vi "calculate_coolprop.vi"(4 "InputCode":T2(ring), 5 "error in":errorcluster, 6 "Input_2":dbl=-1111111111.0 format="%#.6f", 7 "Input_1":dbl=-1111111111.0 format="%#.6f", 8 "Common In":T1={"units"=enum."SI", "Coolprop Directory"=path "C:/Labview/Libfolder/CoolProp.dll", "FluidName"="Water", "Molecular mass [kg/kmol]"=0.0, "Quality [-]"=0.0, "Temperature [°C]"=0.0, "Pressure [bar]"=0.0, "Density [kg/m3]"=0.0, "Spec. heat - ideal gas @ cst. pressure [kJ/kg]"=0.0, "Spec. heat @ cst. pressure [kJ/kg]"=0.0, "Spec. heat @ cst. volume [kJ/kg]"=0.0, "Internal energy [ kJ/kg]"=0.0, "Enthalpy [kJ/kg]"=0.0, "Entropy [kJ/kg-K]"=0.0, "Speed of sound [m/s]"=0.0, "Gibbs function [kJ/kg]"=0.0, "Dynamic viscosity [Pa-s]"=0.0, "Thermal conductivity [kW/m-K]"=0.0, "Surface Tension [N/m]"=0.0, "Accentric factor [-]"=0.0}) -> (0 "error out":errorcluster, 3 "Common Out":T1)   [LabVIEW 2017]
doc: "Calculates thermodynamic values of a certain point for the given fluid, gathered in \"Common Out\".\nCommon connection and InputCode are required.\nIf an input value remains unconnected, the corresponding value in the common will be used.\n\nInput_1 corresponds with the first parameter chosen with the input code.\nInput_2 corresponds with the second parameter chosen with the input code.\ne.g.: if input code is \"TP\", Input_1 requires a temperature (°C) and Input_2 required a pressure (bar)\n\n---\nDesigned by Department of Industrial System and Product Design, Ghent University.\nContact: sergei.gusev@ugent.be; jan.nolens@ugent.be\n\nBased on a Labview-Refprop Wrapper downloaded from Nist.org\nMore info: ken_pop@tom.com yan.ding@jci.com"
uses:
  FluidCommon.ctl
panel:
  out "Array":dbl[](array[numeric])
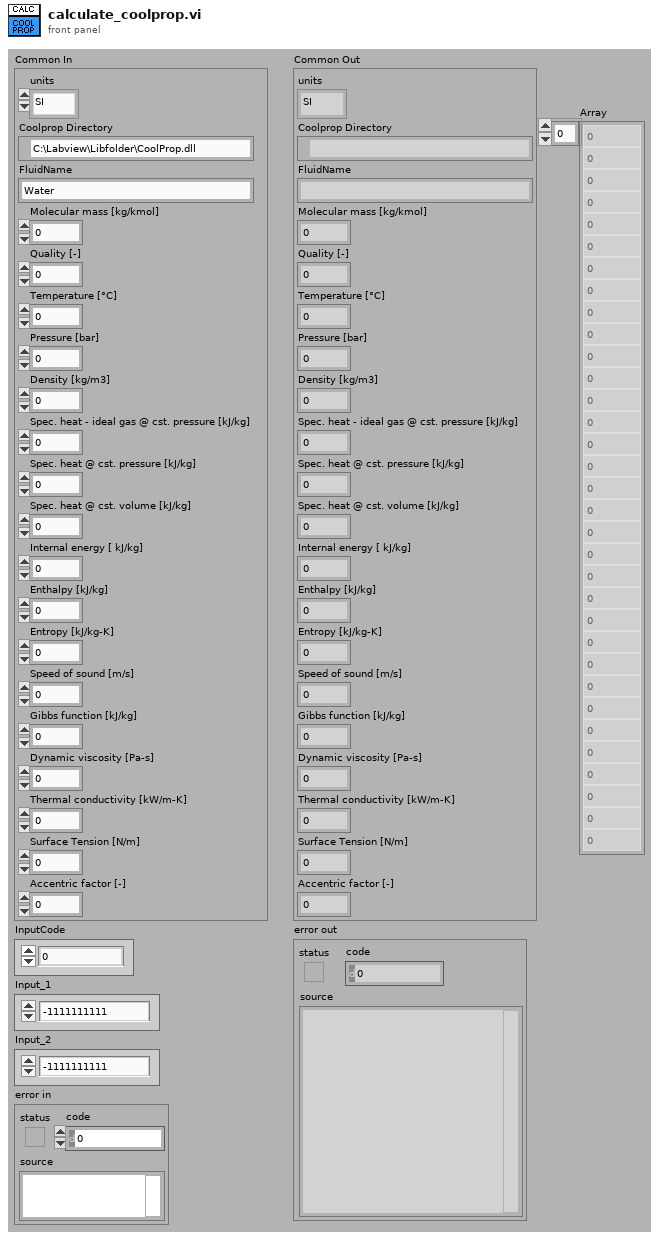
[diagram p1: front panel]
types:
  T1 = typedef "FluidCommon.ctl" = cluster{"units":enum16{"SI", "IP"}, "Coolprop Directory":path, "FluidName":string, "Molecular mass [kg/kmol]":dbl, "Quality [-]":dbl, "Temperature [°C]":dbl, "Pressure [bar]":dbl, "Density [kg/m3]":dbl, "Spec. heat - ideal gas @ cst. pressure [kJ/kg]":dbl, "Spec. heat @ cst. pressure [kJ/kg]":dbl, "Spec. heat @ cst. volume [kJ/kg]":dbl, "Internal energy [ kJ/kg]":dbl, "Enthalpy [kJ/kg]":dbl, "Entropy [kJ/kg-K]":dbl, "Speed of sound [m/s]":dbl, "Gibbs function [kJ/kg]":dbl, "Dynamic viscosity [Pa-s]":dbl, "Thermal conductivity [kW/m-K]":dbl, "Surface Tension [N/m]":dbl, "Accentric factor [-]":dbl}
  T2 = enum16{"0", "TP", "TD", "PD", "TQ", "PQ", "HP", "SP", "SH"}
  T3 = enum16{"P [kPa]", "T [K]", "S [kJ/kg/K]", "H [kJ/kg]"}
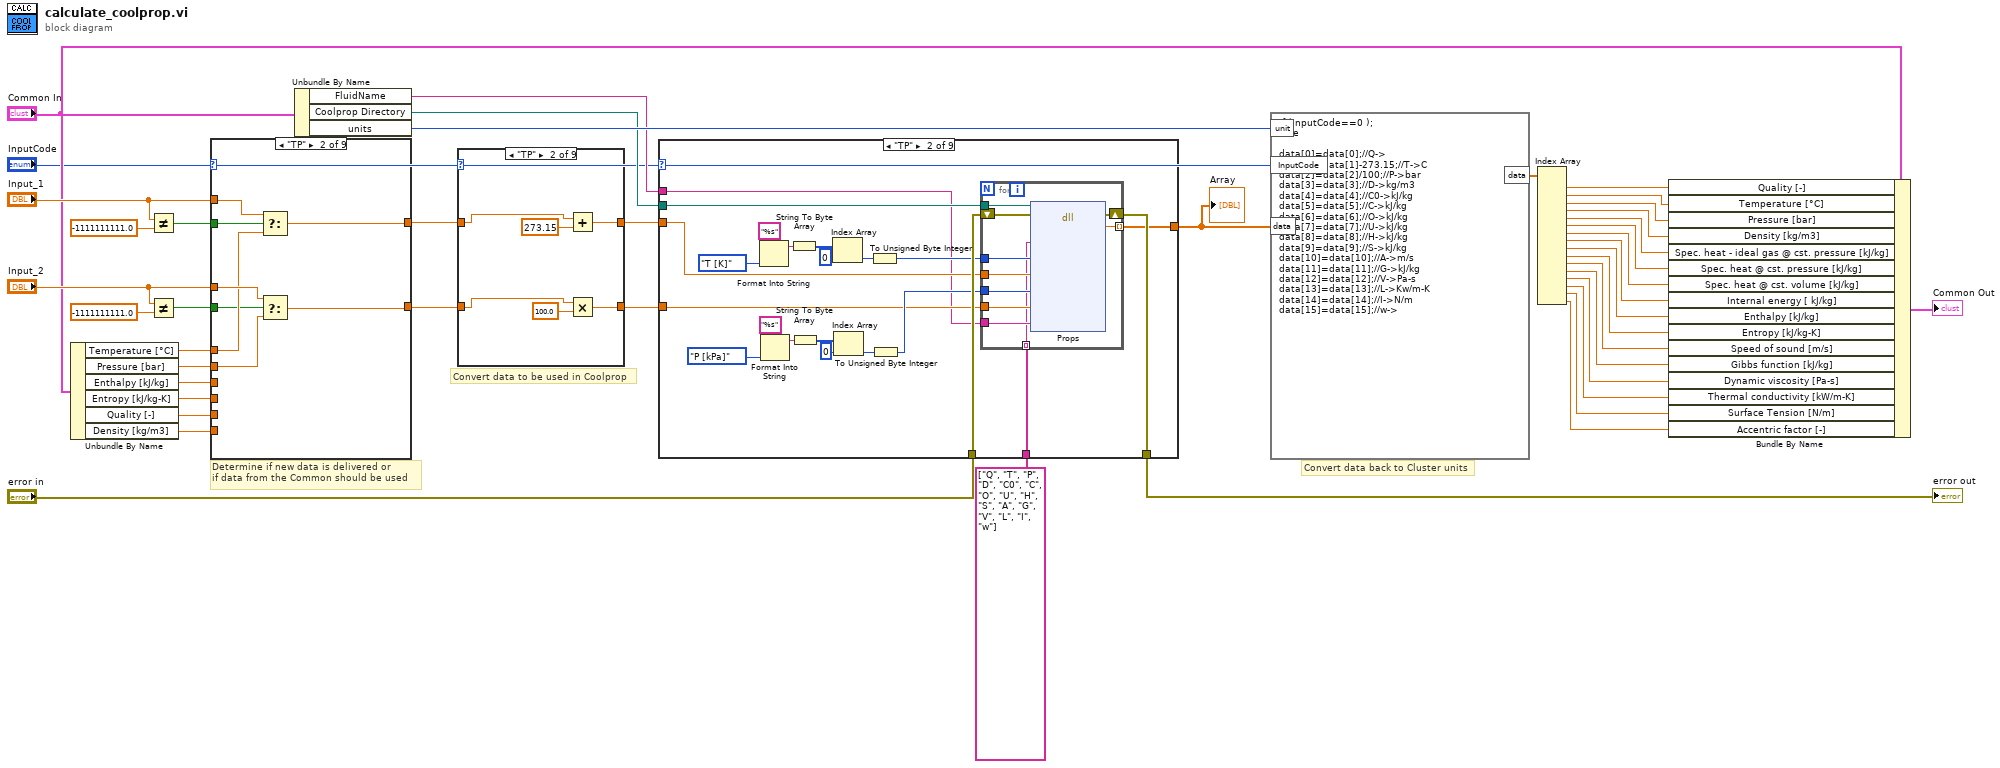
[diagram p0: block diagram]
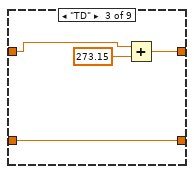
[diagram p3: hidden frame]
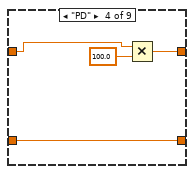
[diagram p4: hidden frame]
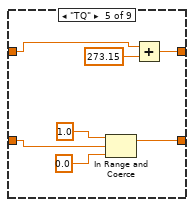
[diagram p5: hidden frame]
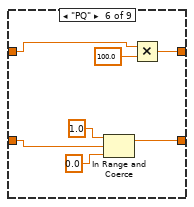
[diagram p6: hidden frame]
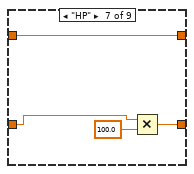
[diagram p7: hidden frame]
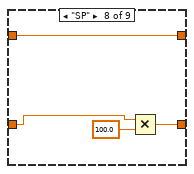
[diagram p8: hidden frame]
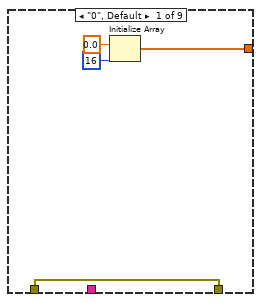
[diagram p10: hidden frame]
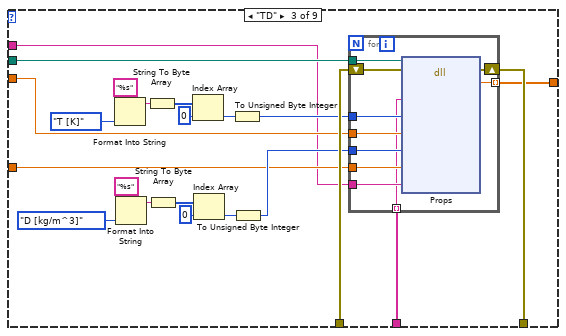
[diagram p11: hidden frame]
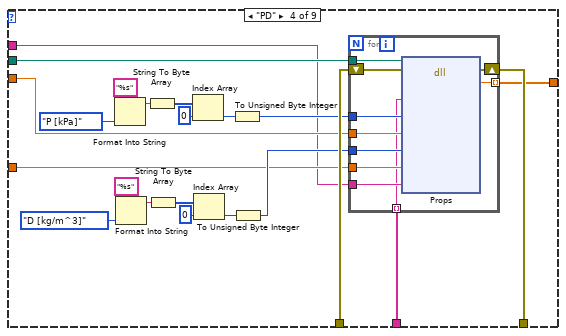
[diagram p12: hidden frame]
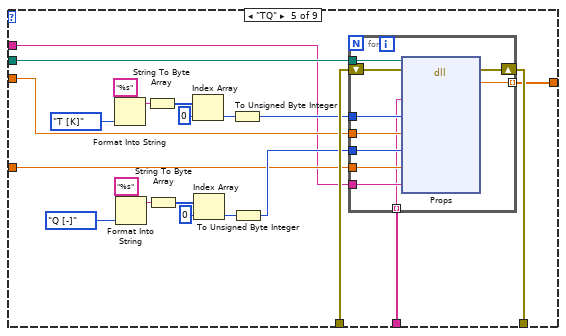
[diagram p13: hidden frame]
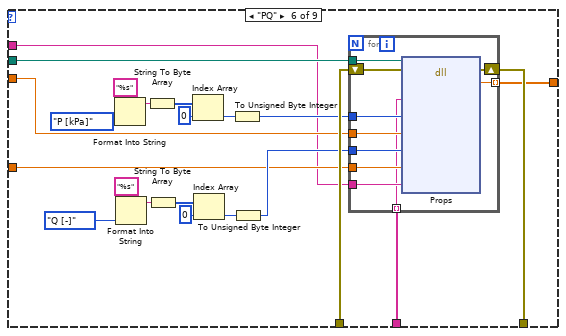
[diagram p14: hidden frame]
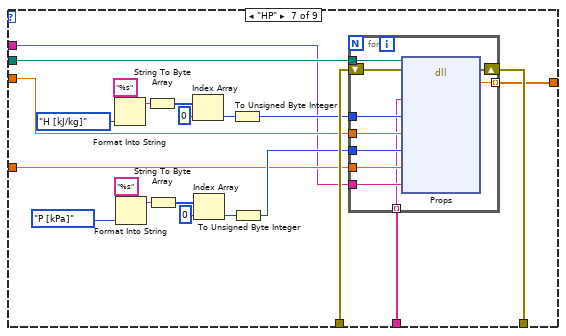
[diagram p15: hidden frame]
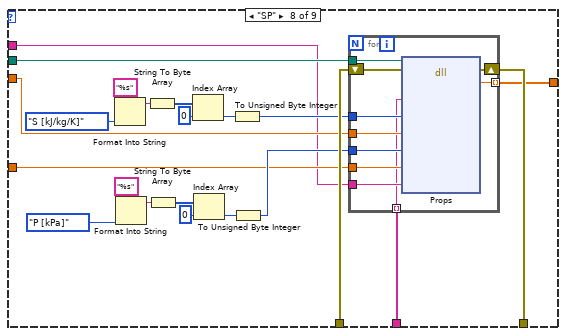
[diagram p16: hidden frame]
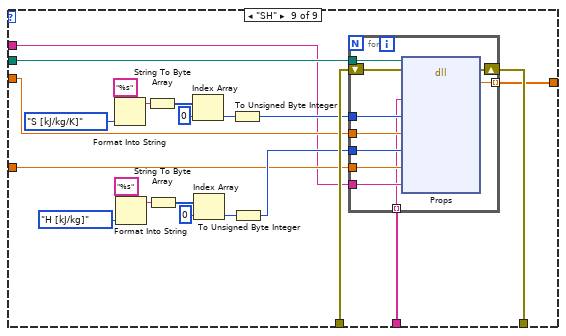
[diagram p17: hidden frame]
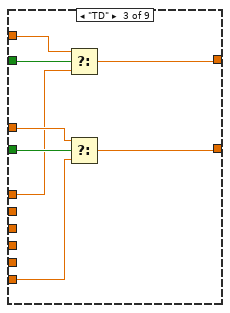
[diagram p19: hidden frame]
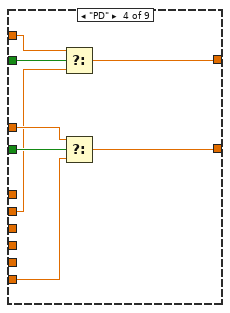
[diagram p20: hidden frame]
diagram:
  # "Convert data back to Cluster units"
  # "Convert data to be used in Coolprop"
  # "Determine if new data is delivered or \nif data from the Common should be used"
  n1 = Unbundle By Name("Common In") -> ("Temperature [°C]"=w35:dbl, "Pressure [bar]"=w34:dbl, "Enthalpy [kJ/kg]"=w33:dbl, "Entropy [kJ/kg-K]"=w32:dbl, "Quality [-]"=w31:dbl, "Density [kg/m3]"=w30:dbl)
  n2 = Not Equal?(x="Input_1", y=-1111111111.0) -> (x != y?=w39:bool)
  n3 = Not Equal?(x="Input_2", y=-1111111111.0) -> (x != y?=w38:bool)
  n4 = case shown="\"TP\"" "InputCode" {
    tunnel: "Input_1" -> [w45 w51 w59 w69 w77 w85 w90 w101 w109]
    tunnel: "Input_2" -> [w44 w53 w57 w67 w75 w83 w92 w99 w107]
    tunnel: w39 -> [_ w49 w58 w68 w76 w84 w91 w100 w108]
    tunnel: w38 -> [_ w48 w56 w66 w74 w82 w93 w98 w106]
    tunnel: w35 -> [_ w50 w55 _ w73 _ _ _ _]
    tunnel: w34 -> [_ w52 _ w65 _ w81 w88 w96 _]
    tunnel: w33 -> [_ _ _ _ _ _ w89 _ w104]
    tunnel: w32 -> [_ _ _ _ _ _ _ w97 w105]
    tunnel: w31 -> [_ _ _ _ w72 w80 _ _ _]
    tunnel: w30 -> [_ _ w54 w64 _ _ _ _ _]
    tunnel: [w45 w47 w60 w62 w70 w78 w86 w94 w102] -> w37
    tunnel: [w44 w46 w61 w63 w71 w79 w87 w95 w103] -> w36
    frame "0", Default {
    }
    frame "TP" {
      n5 = Select(t=w51, s=w49, f=w50) -> (s? t:f=w47:dbl)
      n6 = Select(t=w53, s=w48, f=w52) -> (s? t:f=w46:dbl)
    }
    frame "TD" {
      n7 = Select(t=w59, s=w58, f=w55) -> (s? t:f=w60:dbl)
      n8 = Select(t=w57, s=w56, f=w54) -> (s? t:f=w61:dbl)
    }
    frame "PD" {
      n9 = Select(t=w69, s=w68, f=w65) -> (s? t:f=w62:dbl)
      n10 = Select(t=w67, s=w66, f=w64) -> (s? t:f=w63:dbl)
    }
    frame "TQ" {
      n11 = Select(t=w77, s=w76, f=w73) -> (s? t:f=w70:dbl)
      n12 = Select(t=w75, s=w74, f=w72) -> (s? t:f=w71:dbl)
    }
    frame "PQ" {
      n13 = Select(t=w85, s=w84, f=w81) -> (s? t:f=w78:dbl)
      n14 = Select(t=w83, s=w82, f=w80) -> (s? t:f=w79:dbl)
    }
    frame "HP" {
      n15 = Select(t=w90, s=w91, f=w89) -> (s? t:f=w86:dbl)
      n16 = Select(t=w92, s=w93, f=w88) -> (s? t:f=w87:dbl)
    }
    frame "SP" {
      n17 = Select(t=w101, s=w100, f=w97) -> (s? t:f=w94:dbl)
      n18 = Select(t=w99, s=w98, f=w96) -> (s? t:f=w95:dbl)
    }
    frame "SH" {
      n19 = Select(t=w109, s=w108, f=w105) -> (s? t:f=w102:dbl)
      n20 = Select(t=w107, s=w106, f=w104) -> (s? t:f=w103:dbl)
    }
  }
  n21 = Unbundle By Name("Common In") -> ("FluidName"=w20:string, "Coolprop Directory"=w22:path, "units"=w29:enum16{"SI", "IP"})
  n22 = case shown="\"TP\"" "InputCode" {
    tunnel: [w111 w113 w119 w123 w131 w134 w140 w147 w149] -> w26
    tunnel: w37 -> [w111 w116 w120 w122 w130 w135 w140 w147 w149]
    tunnel: w36 -> [w110 w114 w118 w125 w127 w136 w141 w145 w148]
    tunnel: [w110 w112 w118 w125 w126 w133 w142 w144 w148] -> w25
    frame "0", Default {
    }
    frame "TP" {
      n23 = Add(x=w116, y=273.15) -> (x+y=w113:dbl)
      n24 = Multiply(x=w114, y=100.0 ("x")) -> (x*y=w112:dbl)
    }
    frame "TD" {
      n25 = Add(x=w120, y=273.15) -> (x+y=w119:dbl)
    }
    frame "PD" {
      n26 = Multiply(x=w122, y=100.0 ("x")) -> (x*y=w123:dbl)
    }
    frame "TQ" {
      n27 = In Range and Coerce(upper limit=1.0 ("上限"), x=w127, lower limit=0.0 ("下限")) -> (coerced(x)=w126:dbl)  [unwired: 1 out]
      n28 = Add(x=w130, y=273.15 ("x")) -> (x+y=w131:dbl)
    }
    frame "PQ" {
      n29 = In Range and Coerce(upper limit=1.0 ("上限"), x=w136, lower limit=0.0 ("下限")) -> (coerced(x)=w133:dbl)  [unwired: 1 out]
      n30 = Multiply(x=w135, y=100.0 ("x")) -> (x*y=w134:dbl)
    }
    frame "HP" {
      n31 = Multiply(x=w141, y=100.0 ("x")) -> (x*y=w142:dbl)
    }
    frame "SP" {
      n32 = Multiply(x=w145, y=100.0 ("x")) -> (x*y=w144:dbl)
    }
    frame "SH" {
    }
  }
  n33 = case shown="\"TP\"" "InputCode" {
    tunnel: w26 -> [_ w156 w189 w221 w253 w285 w317 w349 w380]
    tunnel: w25 -> [_ w157 w190 w222 w254 w286 w318 w350 w381]
    tunnel: "error in" -> [w153 w174 w206 w238 w270 w302 w334 w366 w398]
    tunnel: [w153 w173 w205 w237 w269 w301 w333 w365 w397] -> w23
    tunnel: w22 -> [_ w175 w207 w239 w271 w303 w335 w367 w399]
    tunnel: [w150 w172 w204 w236 w268 w300 w332 w364 w396] -> w21
    tunnel: w20 -> [_ w155 w188 w220 w252 w284 w316 w348 w379]
    tunnel: string[] ["Q", "T", "P", "D", "C0", "C", "O", "U", "H", "S", "A", "G", "V", "L", "I", "w"] -> [_ w154 w187 w219 w251 w283 w315 w347 w378]
    frame "0", Default {
      n34 = Initialize Array(0.0 ("元素"), 16 ("维数大小")) -> (w150:dbl[])
    }
    frame "TP" {
      n35 = Format Into String "Format Into String"(format string="%s", T3."T [K]" ("Input Variable #1")) -> (resulting string=w167:string)  [unwired: 2 in, 1 out]
      n36 = Format Into String(format string="%s", T3."P [kPa]" ("Input Variable #1")) -> (resulting string=w161:string)  [unwired: 2 in, 1 out]
      n37 = String To Byte Array(string=w167) -> (unsigned byte array=w169:u8[])
      n38 = String To Byte Array(string=w161) -> (unsigned byte array=w163:u8[])
      n39 = Index Array(array=w169, index=0) -> (element=w171:u8)
      n40 = Index Array(array=w163, index=0) -> (element=w165:u8)
      n41 = To Unsigned Byte Integer(number=w171) -> (unsigned 8bit integer=w159:u8)
      n42 = To Unsigned Byte Integer(number=w165) -> (unsigned 8bit integer=w158:u8)
      n43 = for {
        tunnel: w175 -> [w185]
        shift-right: [w183] -> w173
        shift-left: w174 -> [w184]
        tunnel: [w182] -> w172 mode=indexing
        tunnel: w155 -> [w181]
        tunnel: w157 -> [w180]
        tunnel: w158 -> [w179]
        tunnel: w156 -> [w178]
        tunnel: w159 -> [w177]
        tunnel: w154 -> [w176] mode=indexing
        n44 = dll-call lib="C:/LABVIEW/LibFolder/CoolProp.dll" fn="Props"(path in=w185, error in=w184, "Output"=w176, "Input1"=w177, "Value1"=w178, "Input2"=w179, "Value2"=w180, "Fluid"=w181) -> (error out=w183:errorcluster, "OutputValue"=w182:dbl)  [unwired: 7 in, 1 out]
      }
    }
    frame "TD" {
      n45 = Format Into String "Format Into String"(format string="%s", T3."T [K]" ("Input Variable #1")) -> (resulting string=w199:string)  [unwired: 2 in, 1 out]
      n46 = Format Into String(format string="%s", enum16{"P [kPa]", "Q [-]", "D [kg/m^3]"}."D [kg/m^3]" ("Input Variable #2")) -> (resulting string=w193:string)  [unwired: 2 in, 1 out]
      n47 = String To Byte Array(string=w199) -> (unsigned byte array=w201:u8[])
      n48 = String To Byte Array(string=w193) -> (unsigned byte array=w195:u8[])
      n49 = Index Array(array=w201, index=0) -> (element=w203:u8)
      n50 = Index Array(array=w195, index=0) -> (element=w197:u8)
      n51 = To Unsigned Byte Integer(number=w203) -> (unsigned 8bit integer=w192:u8)
      n52 = To Unsigned Byte Integer(number=w197) -> (unsigned 8bit integer=w191:u8)
      n53 = for {
        tunnel: w207 -> [w217]
        shift-right: [w215] -> w205
        shift-left: w206 -> [w216]
        tunnel: [w214] -> w204 mode=indexing
        tunnel: w188 -> [w213]
        tunnel: w190 -> [w212]
        tunnel: w191 -> [w211]
        tunnel: w189 -> [w210]
        tunnel: w192 -> [w209]
        tunnel: w187 -> [w208] mode=indexing
        n54 = dll-call lib="C:/Coolprop/CoolProp.dll" fn="Props"(path in=w217, error in=w216, "Output"=w208, "Input1"=w209, "Value1"=w210, "Input2"=w211, "Value2"=w212, "Fluid"=w213) -> (error out=w215:errorcluster, "OutputValue"=w214:dbl)  [unwired: 7 in, 1 out]
      }
    }
    frame "PD" {
      n55 = Format Into String "Format Into String"(format string="%s", T3."P [kPa]" ("Input Variable #1")) -> (resulting string=w231:string)  [unwired: 2 in, 1 out]
      n56 = Format Into String(format string="%s", enum16{"P [kPa]", "Q [-]", "D [kg/m^3]"}."D [kg/m^3]" ("Input Variable #2")) -> (resulting string=w225:string)  [unwired: 2 in, 1 out]
      n57 = String To Byte Array(string=w231) -> (unsigned byte array=w233:u8[])
      n58 = String To Byte Array(string=w225) -> (unsigned byte array=w227:u8[])
      n59 = Index Array(array=w233, index=0) -> (element=w235:u8)
      n60 = Index Array(array=w227, index=0) -> (element=w229:u8)
      n61 = To Unsigned Byte Integer(number=w235) -> (unsigned 8bit integer=w224:u8)
      n62 = To Unsigned Byte Integer(number=w229) -> (unsigned 8bit integer=w223:u8)
      n63 = for {
        tunnel: w239 -> [w249]
        shift-right: [w247] -> w237
        shift-left: w238 -> [w248]
        tunnel: [w246] -> w236 mode=indexing
        tunnel: w220 -> [w245]
        tunnel: w222 -> [w244]
        tunnel: w223 -> [w243]
        tunnel: w221 -> [w242]
        tunnel: w224 -> [w241]
        tunnel: w219 -> [w240] mode=indexing
        n64 = dll-call lib="C:/Coolprop/CoolProp.dll" fn="Props"(path in=w249, error in=w248, "Output"=w240, "Input1"=w241, "Value1"=w242, "Input2"=w243, "Value2"=w244, "Fluid"=w245) -> (error out=w247:errorcluster, "OutputValue"=w246:dbl)  [unwired: 7 in, 1 out]
      }
    }
    frame "TQ" {
      n65 = Format Into String "Format Into String"(format string="%s", T3."T [K]" ("Input Variable #1")) -> (resulting string=w263:string)  [unwired: 2 in, 1 out]
      n66 = Format Into String(format string="%s", enum16{"P [kPa]", "Q [-]", "D [kg/m^3]"}."Q [-]" ("Input Variable #2")) -> (resulting string=w257:string)  [unwired: 2 in, 1 out]
      n67 = String To Byte Array(string=w263) -> (unsigned byte array=w265:u8[])
      n68 = String To Byte Array(string=w257) -> (unsigned byte array=w259:u8[])
      n69 = Index Array(array=w265, index=0) -> (element=w267:u8)
      n70 = Index Array(array=w259, index=0) -> (element=w261:u8)
      n71 = To Unsigned Byte Integer(number=w267) -> (unsigned 8bit integer=w256:u8)
      n72 = To Unsigned Byte Integer(number=w261) -> (unsigned 8bit integer=w255:u8)
      n73 = for {
        tunnel: w271 -> [w272]
        shift-right: [w280] -> w269
        shift-left: w270 -> [w281]
        tunnel: [w279] -> w268 mode=indexing
        tunnel: w252 -> [w278]
        tunnel: w254 -> [w277]
        tunnel: w255 -> [w276]
        tunnel: w253 -> [w275]
        tunnel: w256 -> [w274]
        tunnel: w251 -> [w273] mode=indexing
        n74 = dll-call lib="C:/Users/jan.nolens/Desktop/CoolProp.dll" fn="Props"(path in=w272, error in=w281, "Output"=w273, "Input1"=w274, "Value1"=w275, "Input2"=w276, "Value2"=w277, "Fluid"=w278) -> (error out=w280:errorcluster, "OutputValue"=w279:dbl)  [unwired: 7 in, 1 out]
      }
    }
    frame "PQ" {
      n75 = Format Into String "Format Into String"(format string="%s", T3."P [kPa]" ("Input Variable #1")) -> (resulting string=w295:string)  [unwired: 2 in, 1 out]
      n76 = Format Into String(format string="%s", enum16{"P [kPa]", "Q [-]", "D [kg/m^3]"}."Q [-]" ("Input Variable #2")) -> (resulting string=w289:string)  [unwired: 2 in, 1 out]
      n77 = String To Byte Array(string=w295) -> (unsigned byte array=w297:u8[])
      n78 = String To Byte Array(string=w289) -> (unsigned byte array=w291:u8[])
      n79 = Index Array(array=w297, index=0) -> (element=w299:u8)
      n80 = Index Array(array=w291, index=0) -> (element=w293:u8)
      n81 = To Unsigned Byte Integer(number=w299) -> (unsigned 8bit integer=w288:u8)
      n82 = To Unsigned Byte Integer(number=w293) -> (unsigned 8bit integer=w287:u8)
      n83 = for {
        tunnel: w303 -> [w313]
        shift-right: [w311] -> w301
        shift-left: w302 -> [w312]
        tunnel: [w310] -> w300 mode=indexing
        tunnel: w284 -> [w309]
        tunnel: w286 -> [w308]
        tunnel: w287 -> [w307]
        tunnel: w285 -> [w306]
        tunnel: w288 -> [w305]
        tunnel: w283 -> [w304] mode=indexing
        n84 = dll-call lib="C:/Coolprop/CoolProp.dll" fn="Props"(path in=w313, error in=w312, "Output"=w304, "Input1"=w305, "Value1"=w306, "Input2"=w307, "Value2"=w308, "Fluid"=w309) -> (error out=w311:errorcluster, "OutputValue"=w310:dbl)  [unwired: 7 in, 1 out]
      }
    }
    frame "HP" {
      n85 = Format Into String "Format Into String"(format string="%s", T3."H [kJ/kg]" ("Input Variable #1")) -> (resulting string=w327:string)  [unwired: 2 in, 1 out]
      n86 = Format Into String(format string="%s", enum16{"P [kPa]", "Q [-]", "D [kg/m^3]"}."P [kPa]" ("Input Variable #2")) -> (resulting string=w321:string)  [unwired: 2 in, 1 out]
      n87 = String To Byte Array(string=w327) -> (unsigned byte array=w329:u8[])
      n88 = String To Byte Array(string=w321) -> (unsigned byte array=w323:u8[])
      n89 = Index Array(array=w329, index=0) -> (element=w331:u8)
      n90 = Index Array(array=w323, index=0) -> (element=w325:u8)
      n91 = To Unsigned Byte Integer(number=w331) -> (unsigned 8bit integer=w320:u8)
      n92 = To Unsigned Byte Integer(number=w325) -> (unsigned 8bit integer=w319:u8)
      n93 = for {
        tunnel: w335 -> [w345]
        shift-right: [w343] -> w333
        shift-left: w334 -> [w344]
        tunnel: [w342] -> w332 mode=indexing
        tunnel: w316 -> [w341]
        tunnel: w318 -> [w340]
        tunnel: w319 -> [w339]
        tunnel: w317 -> [w338]
        tunnel: w320 -> [w337]
        tunnel: w315 -> [w336] mode=indexing
        n94 = dll-call lib="C:/Coolprop/CoolProp.dll" fn="Props"(path in=w345, error in=w344, "Output"=w336, "Input1"=w337, "Value1"=w338, "Input2"=w339, "Value2"=w340, "Fluid"=w341) -> (error out=w343:errorcluster, "OutputValue"=w342:dbl)  [unwired: 7 in, 1 out]
      }
    }
    frame "SP" {
      n95 = Format Into String "Format Into String"(format string="%s", T3."S [kJ/kg/K]" ("Input Variable #1")) -> (resulting string=w359:string)  [unwired: 2 in, 1 out]
      n96 = Format Into String(format string="%s", enum16{"P [kPa]", "Q [-]", "D [kg/m^3]"}."P [kPa]" ("Input Variable #2")) -> (resulting string=w353:string)  [unwired: 2 in, 1 out]
      n97 = String To Byte Array(string=w359) -> (unsigned byte array=w361:u8[])
      n98 = String To Byte Array(string=w353) -> (unsigned byte array=w355:u8[])
      n99 = Index Array(array=w361, index=0) -> (element=w363:u8)
      n100 = Index Array(array=w355, index=0) -> (element=w357:u8)
      n101 = To Unsigned Byte Integer(number=w363) -> (unsigned 8bit integer=w352:u8)
      n102 = To Unsigned Byte Integer(number=w357) -> (unsigned 8bit integer=w351:u8)
      n103 = for {
        tunnel: w367 -> [w377]
        shift-right: [w375] -> w365
        shift-left: w366 -> [w376]
        tunnel: [w374] -> w364 mode=indexing
        tunnel: w348 -> [w373]
        tunnel: w350 -> [w372]
        tunnel: w351 -> [w371]
        tunnel: w349 -> [w370]
        tunnel: w352 -> [w369]
        tunnel: w347 -> [w368] mode=indexing
        n104 = dll-call lib="C:/Coolprop/CoolProp.dll" fn="Props"(path in=w377, error in=w376, "Output"=w368, "Input1"=w369, "Value1"=w370, "Input2"=w371, "Value2"=w372, "Fluid"=w373) -> (error out=w375:errorcluster, "OutputValue"=w374:dbl)  [unwired: 7 in, 1 out]
      }
    }
    frame "SH" {
      n105 = Format Into String "Format Into String"(format string="%s", T3."S [kJ/kg/K]" ("Input Variable #1")) -> (resulting string=w391:string)  [unwired: 2 in, 1 out]
      n106 = Format Into String(format string="%s", T3."H [kJ/kg]" ("Input Variable #1")) -> (resulting string=w385:string)  [unwired: 2 in, 1 out]
      n107 = String To Byte Array(string=w391) -> (unsigned byte array=w393:u8[])
      n108 = String To Byte Array(string=w385) -> (unsigned byte array=w387:u8[])
      n109 = Index Array(array=w393, index=0) -> (element=w395:u8)
      n110 = Index Array(array=w387, index=0) -> (element=w389:u8)
      n111 = To Unsigned Byte Integer(number=w395) -> (unsigned 8bit integer=w383:u8)
      n112 = To Unsigned Byte Integer(number=w389) -> (unsigned 8bit integer=w382:u8)
      n113 = for {
        tunnel: w399 -> [w409]
        shift-right: [w407] -> w397
        shift-left: w398 -> [w408]
        tunnel: [w406] -> w396 mode=indexing
        tunnel: w379 -> [w405]
        tunnel: w381 -> [w404]
        tunnel: w382 -> [w403]
        tunnel: w380 -> [w402]
        tunnel: w383 -> [w401]
        tunnel: w378 -> [w400] mode=indexing
        n114 = dll-call lib="C:/Coolprop/CoolProp.dll" fn="Props"(path in=w409, error in=w408, "Output"=w400, "Input1"=w401, "Value1"=w402, "Input2"=w403, "Value2"=w404, "Fluid"=w405) -> (error out=w407:errorcluster, "OutputValue"=w406:dbl)  [unwired: 7 in, 1 out]
      }
    }
  }
  "error out" <- w23
  "Array" <- w21
  n115 = formula code="if (InputCode==0 );\nelse\n\ndata[0]=data[0];//Q->\ndata[1]=data[1]-273.15;//T->C\ndata[2]=data[2]/100;//P->bar\ndata[3]=data[3];//D->kg/m3\ndata[4]=data[4];//C0->kJ/kg\ndata[5]=data[5];//C->kJ/kg\ndata[6]=data[6];//O->kJ/kg\ndata[7]=data[7];//U->kJ/kg\ndata[8]=data[8];//H->kJ/kg\ndata[9]=data[9];//S->kJ/kg\ndata[10]=data[10];//A->m/s\ndata[11]=data[11];//G->kJ/kg\ndata[12]=data[12];//V->Pa-s\ndata[13]=data[13];//L->Kw/m-K\ndata[14]=data[14];//I->N/m\ndata[15]=data[15];//w->"("data"=w21, "unit"=w29, "InputCode"="InputCode") -> ("data"=w18:dbl[])
  n116 = Index Array(array=w18) -> (element #1=w17:dbl, element #2=w16:dbl, element #3=w15:dbl, element #4=w14:dbl, element #5=w13:dbl, element #6=w12:dbl, element #7=w11:dbl, element #8=w10:dbl, element #9=w9:dbl, element #10=w8:dbl, element #11=w7:dbl, element #12=w6:dbl, element #13=w5:dbl, element #14=w4:dbl, element #15=w3:dbl, element #16=w2:dbl)  [unwired: 16 in]
  n117 = Bundle By Name(cluster="Common In", "Quality [-]"=w17, "Temperature [°C]"=w16, "Pressure [bar]"=w15, "Density [kg/m3]"=w14, "Spec. heat - ideal gas @ cst. pressure [kJ/kg]"=w13, "Spec. heat @ cst. pressure [kJ/kg]"=w12, "Spec. heat @ cst. volume [kJ/kg]"=w11, "Internal energy [ kJ/kg]"=w10, "Enthalpy [kJ/kg]"=w9, "Entropy [kJ/kg-K]"=w8, "Speed of sound [m/s]"=w7, "Gibbs function [kJ/kg]"=w6, "Dynamic viscosity [Pa-s]"=w5, "Thermal conductivity [kW/m-K]"=w4, "Surface Tension [N/m]"=w3, "Accentric factor [-]"=w2) -> (→"Common Out":T1)
